vi "Send Update Test Node Map Msg.vi"(10 "Mode":string, 11 "Message Enqueuer in":refnum<class "Message Enqueuer.lvclass">) -> (3 "Message Enqueuer out":refnum<class "Message Enqueuer.lvclass">)   [LabVIEW 2013, in "Abstract Messages.lvlib"]
uses:
  Abstract Messages.lvlib
  <vilib>/ActorFramework/Message Enqueuer/Message Enqueuer.lvclass
  Abstract Update Test Node Map Msg.lvclass
  <vilib>/ActorFramework/Message Enqueuer/Message Enqueuer.lvclass/Message Enqueuer.ctl
  <vilib>/ActorFramework/Message Priority Queue/Priority Enqueue.vi
  <vilib>/ActorFrameworkMVC/UI Controller Messages/Get Model Actor Enqueuer Msg/Get Model Actor Enqueuer Msg.lvclass
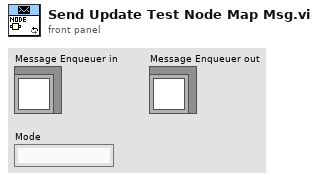
[diagram p1: front panel]
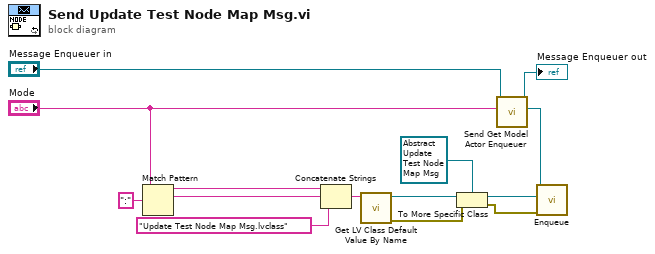
[diagram p0: block diagram]
diagram:
  n1 = Match Pattern(string="Mode", regular expression=":") -> (before substring=w10:string, match substring=w11:string)  [unwired: 1 in, 2 out]
  n2 = Concatenate Strings(w10, w11, "Update Test Node Map Msg.lvclass" ("element")) -> (w12:string)
  n3 = call <vilib>:"Get LV Class Default Value By Name.vi"("class name"=w12) -> ("error out"=w1:errorcluster, "object"=w8:refnum<class>)  [unwired: 9 in]
  n4 = To More Specific Class(target class=refnum<class "Abstract Update Test Node Map Msg.lvclass"> refnum ("Abstract Messages.lvlib:Abstract Update Test Node Map Msg.lvclass"), reference=w8, error in=w1) -> (specific class reference=w13:refnum<class "Abstract Update Test Node Map Msg.lvclass">, error out=w2:errorcluster)
  n5 = call <vilib>:"Send Get Model Actor Enqueuer.vi"("Model Name"="Mode", "Message Enqueuer in"="Message Enqueuer in") -> ("Reply"=w3:refnum<class "Message Enqueuer.lvclass">, "Message Enqueuer out"=→"Message Enqueuer out":refnum<class "Message Enqueuer.lvclass">)  [unwired: 6 in, 2 out]
  n6 = call <vilib>:"Enqueue.vi"("error in (no error)"=w2, "Message"=w13, "Message Enqueuer in"=w3) -> ()  [unwired: 7 in, 2 out]
